vi "CCD photon image_Shaowei-v3.vi"() -> ()   [LabVIEW 2009]
uses:
  <vilib>/Utility/file.llb/Read From Spreadsheet File (DBL).vi
  Instance           5 35Saved   CCD photon image_540_800_CR .vi
  Instance           4 35Saved   CCD photon image_540_800_CR .vi
  Instance           3 35Saved   CCD photon image_540_800_CR .vi
  Instance           8 35Saved   CCD photon image_540_800_CR .vi
  <vilib>/Analysis/Matrix/Numeric/Conversions/Array To Matrix - RA2.vi
  Instance          12 35Saved   CCD photon image_540_800_CR .vi
  Instance          18 35Saved   CCD photon image_540_800_CR .vi
  <vilib>/Analysis/Matrix/NI_Matrix.lvlib
panel:
  in  "Full Range 5":bool caption="Full Range"
  in  "Full Range 4":bool caption="Full Range"
  in  "Full Range":bool
  in  "Full Range 3":bool caption="Full Range"
  in  "Full Range":bool
  in  "Full Range":bool
  in  "Save Matrix6":bool
  in  "Save Matrix5":bool
  in  "Save Matrix3":bool
  in  "Save Matrix4":bool
  out "Save As":string
  in  "Save Matrix2":bool
  out "Save As":string
  in  "Save Matrix1":bool
  in  "select 2":bool
  in  "select":bool
  in  "next 2":bool
  in  "next":bool
  in  "previous 2":bool
  in  "previous":bool
  in  "Do it":bool
  out "?":path
  out "?":path
  out "?":i32
  in  "?":bool
  in  "stop 2":bool
  in  "#6":bool
  in  "#5":bool
  in  "to":dbl=950.0
  in  "From":dbl=550.0
  out "Intensity Graph 6":dbl[][](graph)
  out "px":dbl
  out "px":dbl
  out "Save As":string
  in  "From 5":dbl caption="From"
  in  "To 5":dbl caption="To"
  out "eV":dbl format="%#_4g"
  out "eV":dbl format="%#_4g"
  out "Intensity Graph 5":dbl[][](graph)
  out "px":dbl
  out "px":dbl
  out "Save As":string
  in  "From 4":dbl caption="From"
  in  "To 4":dbl caption="To"
  out "eV":dbl format="%#_4g"
  out "eV":dbl format="%#_4g"
  in  "?":bool
  out "MAX":dbl
  out "MIN":dbl
  out "X":sgl
  out "Y":sgl
  out "px":dbl
  out "px":dbl
  out "eV":dbl format="%#_4g"
  out "eV":dbl format="%#_4g"
  in  "To 3":dbl caption="To"
  in  "From 3":dbl caption="From"
  out "eV":dbl format="%#_4g"
  out "eV":dbl format="%#_4g"
  in  "To":dbl
  in  "From":dbl
  out "px":dbl
  out "px":dbl
  out "px":dbl
  out "px":dbl
  out "eV":dbl format="%#_4g"
  out "eV":dbl format="%#_4g"
  in  "To":dbl
  in  "From":dbl
  in  "?":dbl=32.0
  out "eV":dbl format="%#_4g"
  out "eV":dbl format="%#_4g"
  in  "To":dbl
  in  "From":dbl
  out "px":dbl
  out "px":dbl
  in  "#3":bool
  in  "#4":bool
  in  "#2":bool
  out "Intensity Graph 4":dbl[][](graph)
  out "Save As":string
  out "Intensity Graph 3":dbl[][](graph)
  out "Save As":string
  out "Intensity Graph 2":dbl[][](graph)
  out "Intensity Graph":dbl[][](graph)
  # "Input File"
  # "nm"
  # "nm"
  # "nm"
  # "2 Files"
  # "1 File"
  # "nm"
  # "nm"
  # "nm"
  # "1st"
  # "2nd"
  # "Spectra Range"
  # "nm"
  # "nm"
  # "# of Pixel"
  # "Image Size"
  # "Bit"
  # "Active Window"
  # "nm"
  # "nm"
  # "nm"
  # "nm"
  # "nm"
  # "nm"
  # "Cosmic Ray Removal"
  # "NO"
  # "YES"
  # "Value"
  # "Position"
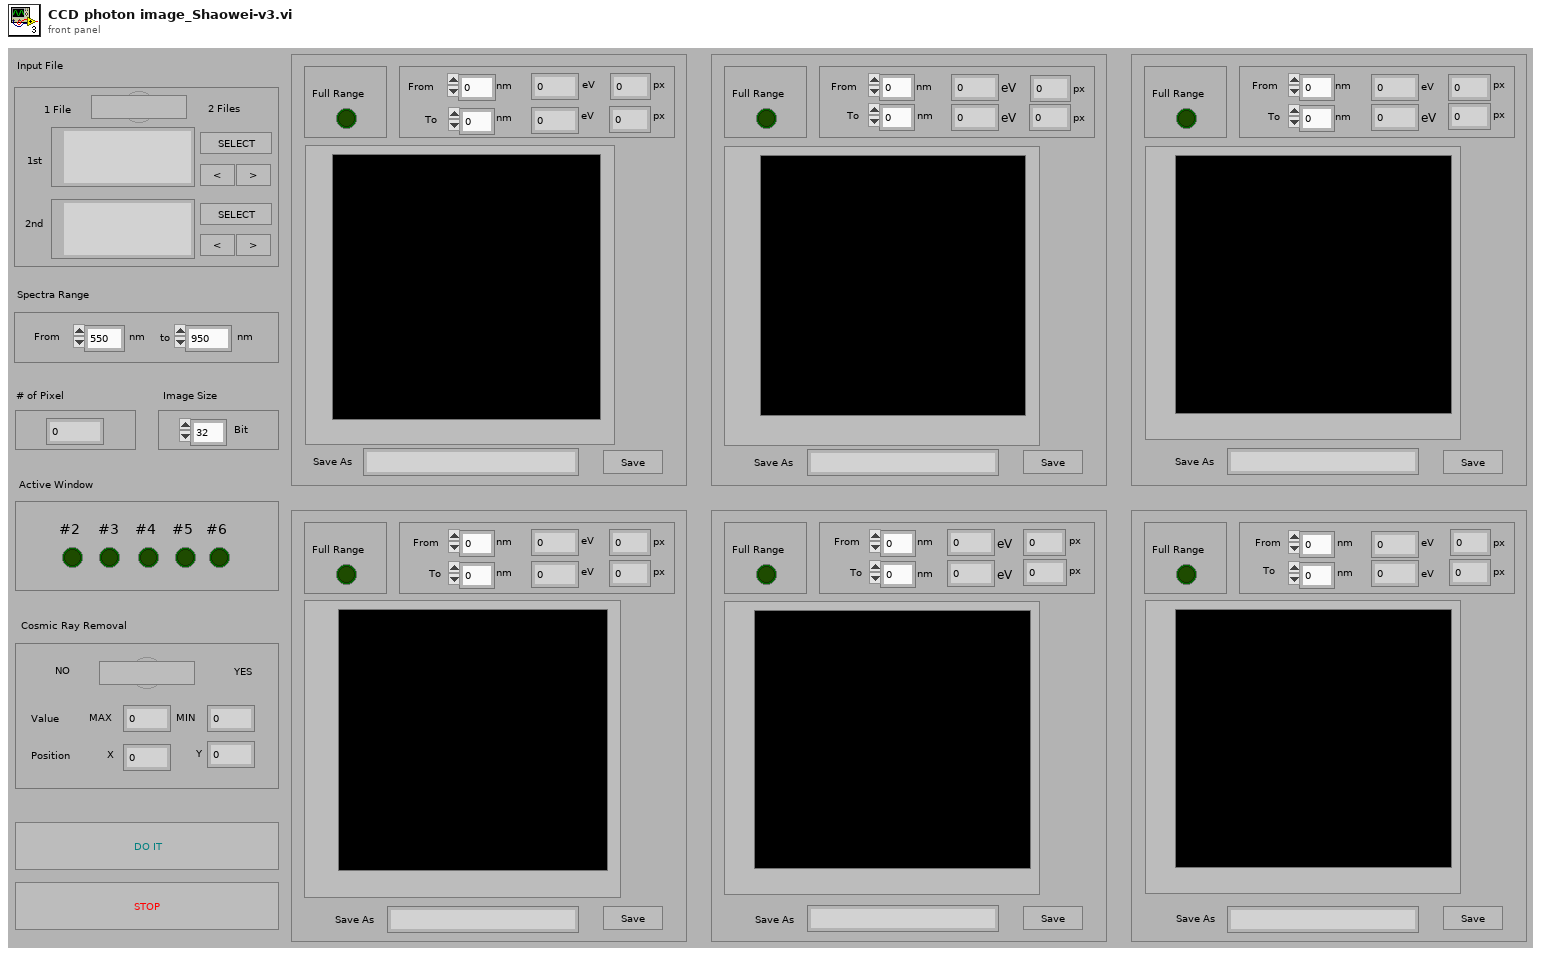
[diagram p1: front panel]
types:
  T1 = typedef "NI_Matrix.lvlib/RealMatrix.ctl" = dbl[][]
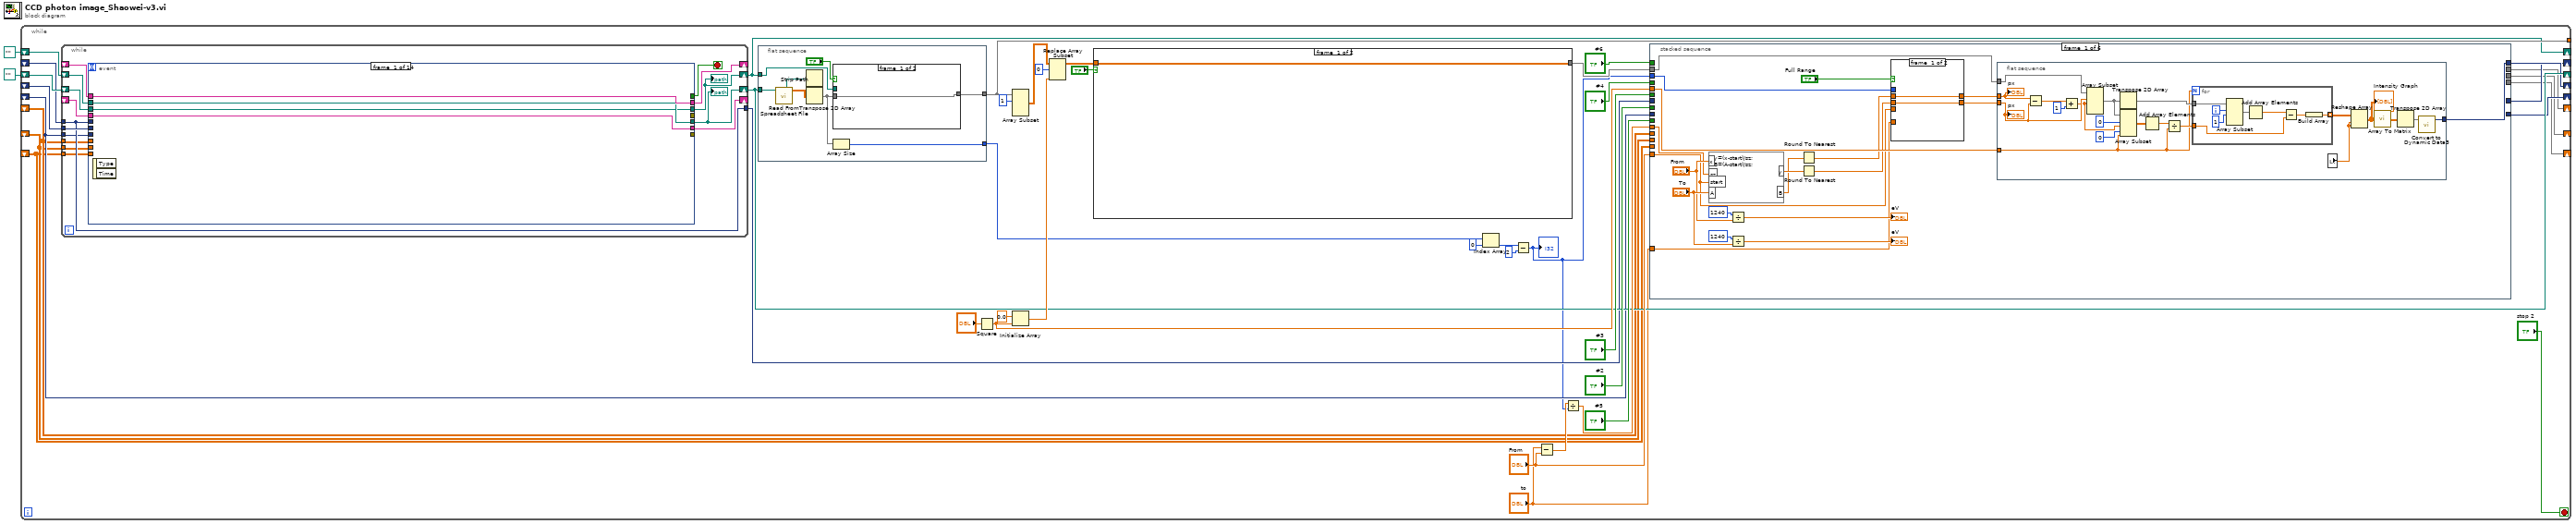
[diagram p0: block diagram]
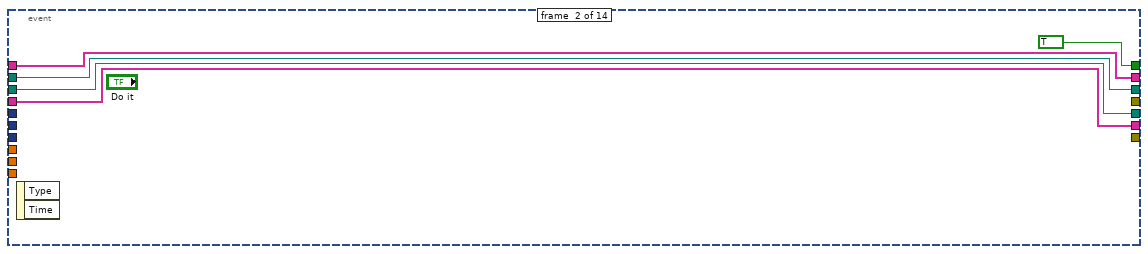
[diagram p2: hidden frame]
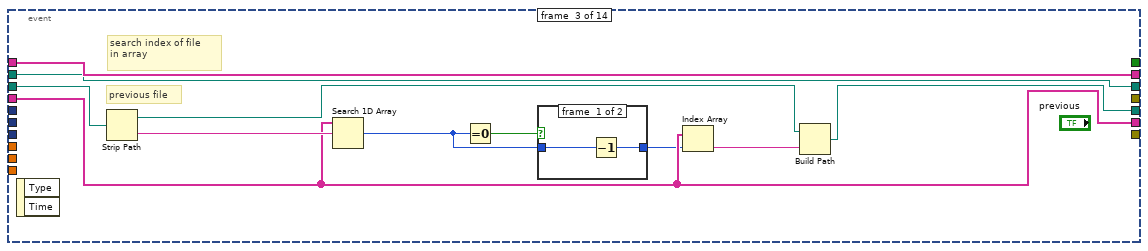
[diagram p3: hidden frame]
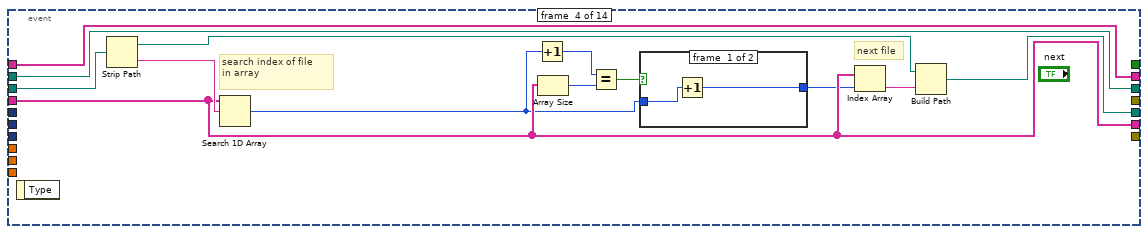
[diagram p5: hidden frame]
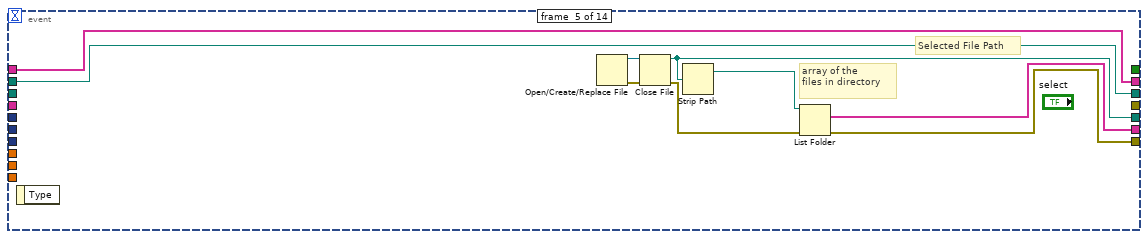
[diagram p7: hidden frame]
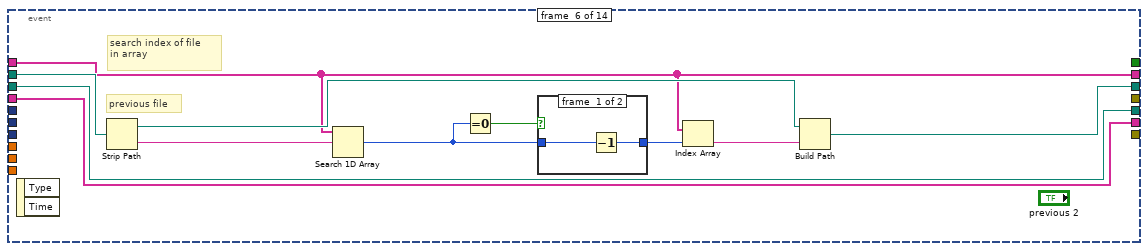
[diagram p8: hidden frame]
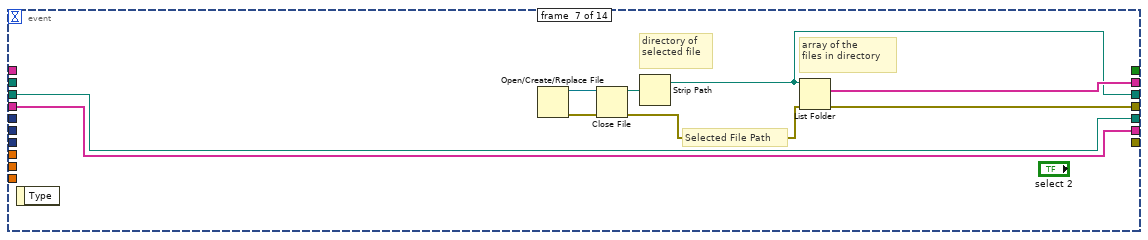
[diagram p10: hidden frame]
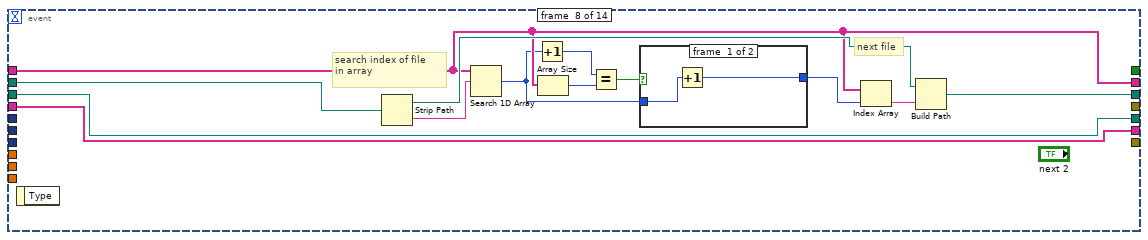
[diagram p11: hidden frame]
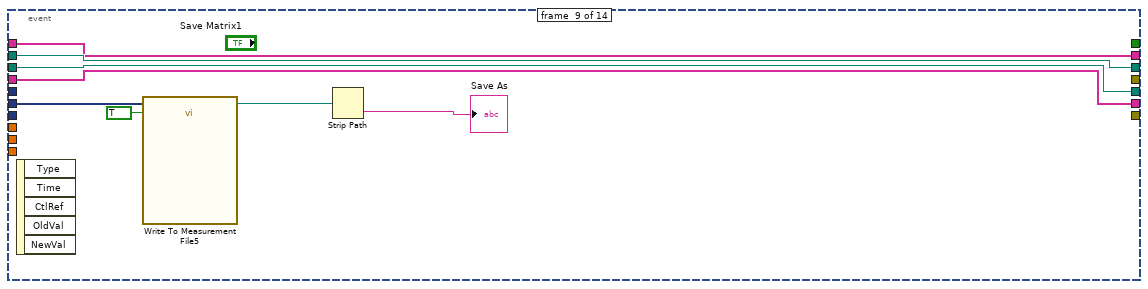
[diagram p13: hidden frame]
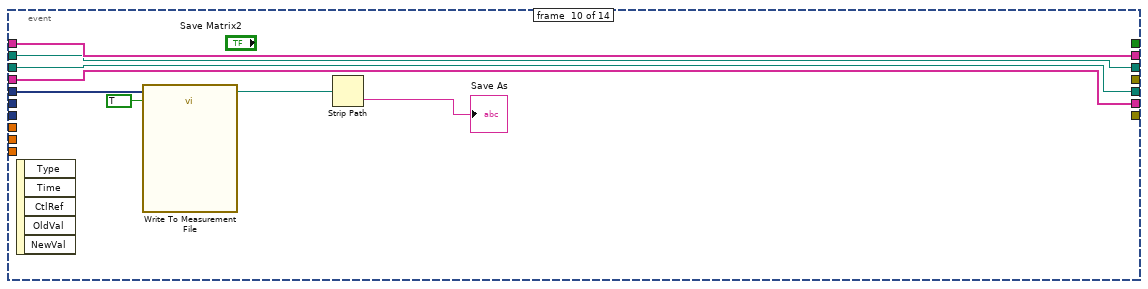
[diagram p14: hidden frame]
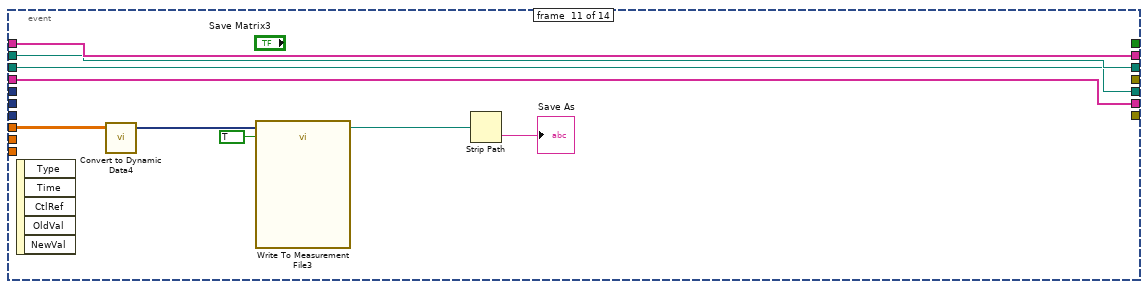
[diagram p15: hidden frame]
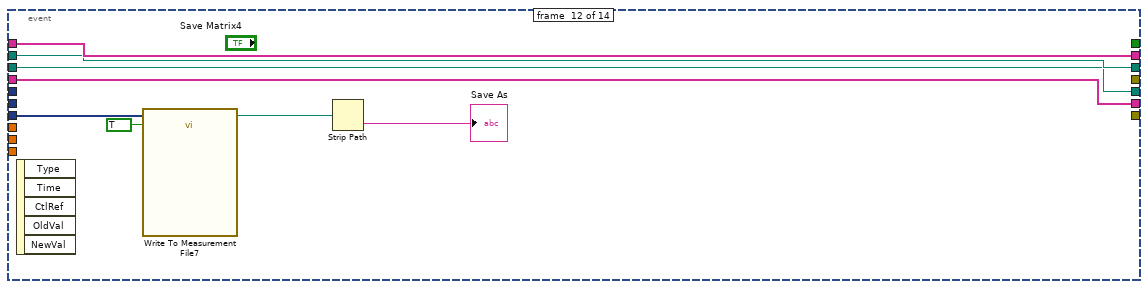
[diagram p16: hidden frame]
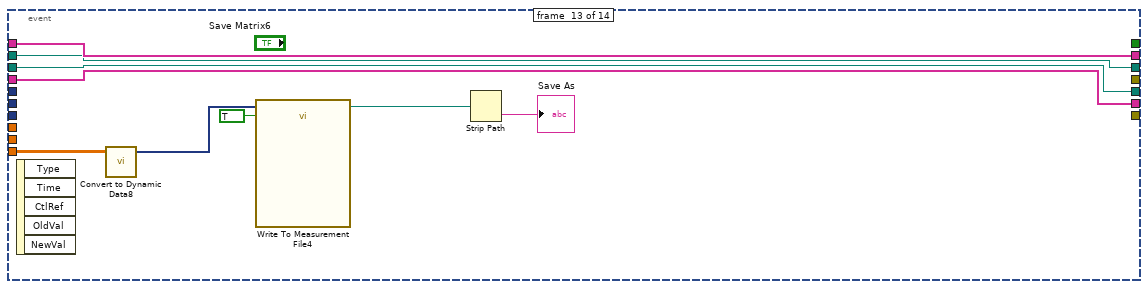
[diagram p17: hidden frame]
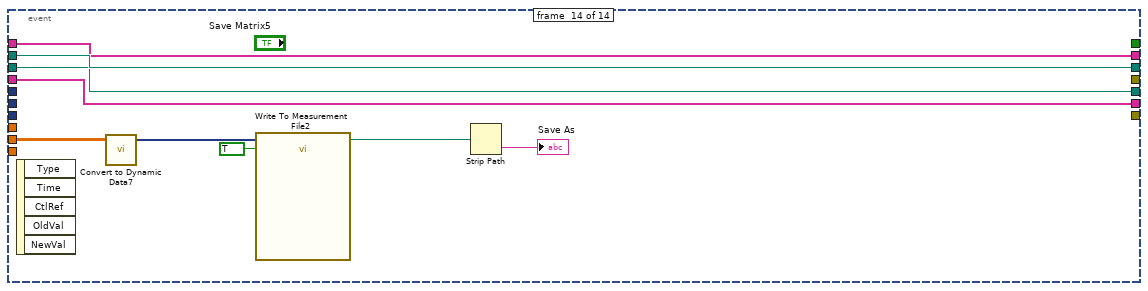
[diagram p18: hidden frame]
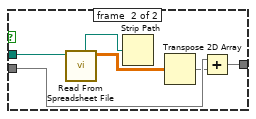
[diagram p19: hidden frame]
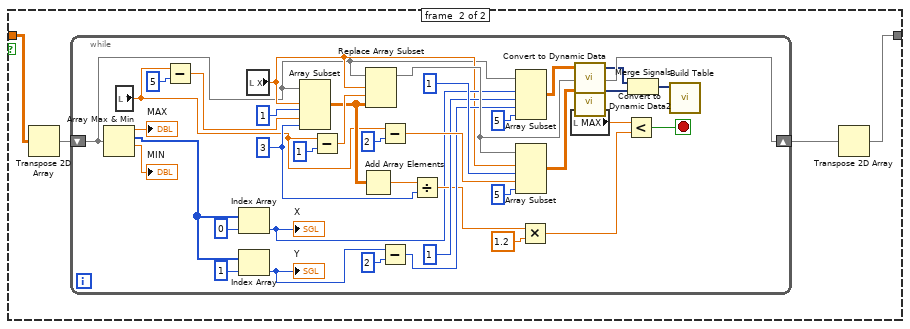
[diagram p20: hidden frame]
diagram:
  n1 = while {
    tunnel: [w27] -> _
    shift-right: [w18] -> _
    shift-left: path "" ("path") -> [w20]
    shift-right: [w19] -> _
    shift-left: path "" ("path") -> [w21]
    shift-right: [w17] -> _
    shift-left: _ -> [w16]
    shift-right: [w15] -> _
    shift-left: _ -> [w14]
    shift-right: [w12] -> _
    shift-left: _ -> [w11]
    shift-right: [w10] -> _
    shift-left: _ -> [w9]
    shift-right: [w8] -> _
    shift-left: _ -> [w7]
    shift-right: [w6] -> _
    shift-left: _ -> [w5]
    stop <- "stop 2" stop-if-true
    n2 = while {
      shift-right: [w60] -> _
      shift-left: _ -> [w59]
      shift-right: [w46] -> w18
      shift-left: w20 -> [w58]
      shift-right: [w47] -> w19
      shift-left: w21 -> [w57]
      shift-right: [w56] -> _
      shift-left: _ -> [w55]
      tunnel: w16 -> [w53]
      tunnel: w14 -> [w52]
      tunnel: [w52] -> w13
      tunnel: w11 -> [w51]
      tunnel: w9 -> [w50]
      tunnel: w7 -> [w49]
      tunnel: w5 -> [w48]
      stop <- w54 stop-if-true
      n3 = event shown="[1] \"Do it\": Value Change" {
        selector: _ -> [_ _ _ _ _ _ _ _ _ _ _ _ _ _]
        dyn-events: _ -> [_ _ _ _ _ _ _ _ _ _ _ _ _ _]
        timeout: _ -> [_ _ _ _ _ _ _ _ _ _ _ _ _ _]
        tunnel: [_ TRUE _ _ _ _ _ _ _ _ _ _ _ _] -> w54
        tunnel: [w63 w68 w75 w93 w103 w109 w130 w139 w151 w157 w165 w174 w182 w190] -> w46
        tunnel: [w64 w69 w77 w89 w107 w114 w129 w138 w148 w156 w164 w173 w181 w191] -> w60
        tunnel: w59 -> [w64 w69 w77 w89 _ w114 w129 w138 w148 w156 w164 w173 w181 w191]
        tunnel: w58 -> [w63 w68 w80 w92 _ w109 w130 w139 w151 w157 w165 w174 w182 w190]
        tunnel: [w61 w66 w73 w90 w105 w110 w128 w140 w150 w158 w166 w175 w183 w193] -> w47
        tunnel: w57 -> [w61 w66 w73 w90 w105 w116 _ w141 w150 w158 w166 w175 w183 w193]
        tunnel: [w62 w67 w74 w91 w106 w115 w131 w134 w149 w159 w167 w176 w184 w192] -> w56
        tunnel: w55 -> [w62 w67 w74 w91 w106 w115 _ w134 w149 w159 w167 w176 w184 w192]
        tunnel: w53 -> [_ _ _ _ _ _ _ _ w155 _ _ _ _ _]
        tunnel: w52 -> [_ _ _ _ _ _ _ _ _ w163 _ _ _ _]
        tunnel: w51 -> [_ _ _ _ _ _ _ _ _ _ _ w177 _ _]
        tunnel: w50 -> [_ _ _ _ _ _ _ _ _ _ w169 _ _ _]
        tunnel: w49 -> [_ _ _ _ _ _ _ _ _ _ _ _ _ w196]
        tunnel: w48 -> [_ _ _ _ _ _ _ _ _ _ _ _ w186 _]
        tunnel: [_ _ _ _ _ _ w123 _ _ _ _ _ _ _] -> _
        tunnel: [_ _ _ _ w100 _ _ _ _ _ _ _ _ _] -> _
        event #0 {
          n4 = event-data() -> ()  [unwired: 1 in, 2 out]
        }
        event #1 {
          n5 = event-data() -> ()  [unwired: 1 in, 2 out]
        }
        event #2 {
          # "previous file"
          # "search index of file\nin array"
          n6 = event-data() -> ()  [unwired: 1 in, 2 out]
          n7 = Strip Path(path=w80) -> (stripped path=w78:path, name=w79:string)
          n8 = Search 1D Array(1D array=w77, element=w79) -> (index of element=w71:i32)  [unwired: 1 in]
          n9 = Equal To 0?(x=w71) -> (x = 0?=w72:bool)
          n10 = case shown="False" w72 {
            tunnel: w71 -> [w82 w83]
            tunnel: [w81 w83] -> w70
            frame #0 {
              n11 = Decrement(x=w82) -> (x-1=w81:i32)
            }
            frame #1 {
            }
          }
          n12 = Index Array(array=w77, index=w70) -> (element=w76:string)
          n13 = Build Path(base path=w78, name or relative path=w76) -> (appended path=w75:path)
        }
        event #3 {
          # "next file"
          # "search index of file\nin array"
          n14 = event-data() -> ()  [unwired: 1 in, 1 out]
          n15 = Strip Path(path=w92) -> (stripped path=w95:path, name=w96:string)
          n16 = Search 1D Array(1D array=w89, element=w96) -> (index of element=w84:i32)  [unwired: 1 in]
          n17 = Increment(x=w84) -> (x+1=w85:i32)
          n18 = Array Size(array=w89) -> (size(s)=w88:i32)
          n19 = Equal?(x=w85, y=w88) -> (x = y?=w87:bool)
          n20 = case shown="True" w87 {
            tunnel: w84 -> [w98 w99]
            tunnel: [w97 w99] -> w86
            frame #0 {
              n21 = Increment(x=w98) -> (x+1=w97:i32)
            }
            frame #1 {
            }
          }
          n22 = Index Array(array=w89, index=w86) -> (element=w94:string)
          n23 = Build Path(base path=w95, name or relative path=w94) -> (appended path=w93:path)
        }
        event #4 {
          # "array of the \nfiles in directory"
          # "Selected File Path"
          n24 = event-data() -> ()  [unwired: 1 in, 1 out]
          n25 = Open/Create/Replace File() -> (refnum out=w104:refnum<file>, error out=w102:errorcluster)  [unwired: 6 in, 1 out]
          n26 = Close File(refnum=w104, error in=w102) -> (path=w103:path, error out=w101:errorcluster)
          n27 = Strip Path(path=w103) -> (stripped path=w108:path)  [unwired: 1 out]
          n28 = List Folder(path=w108, error in=w101) -> (filenames=w107:string[], error out=w100:errorcluster)  [unwired: 2 in, 2 out]
        }
        event #5 {
          # "previous file"
          # "search index of file\nin array"
          n29 = event-data() -> ()  [unwired: 1 in, 2 out]
          n30 = Strip Path(path=w116) -> (stripped path=w118:path, name=w119:string)
          n31 = Search 1D Array(1D array=w115, element=w119) -> (index of element=w112:i32)  [unwired: 1 in]
          n32 = Equal To 0?(x=w112) -> (x = 0?=w113:bool)
          n33 = case shown="False" w113 {
            tunnel: w112 -> [w121 w122]
            tunnel: [w120 w122] -> w111
            frame #0 {
              n34 = Decrement(x=w121) -> (x-1=w120:i32)
            }
            frame #1 {
            }
          }
          n35 = Index Array(array=w115, index=w111) -> (element=w117:string)
          n36 = Build Path(base path=w118, name or relative path=w117) -> (appended path=w110:path)
        }
        event #6 {
          # "array of the \nfiles in directory"
          # "directory of\nselected file"
          # "Selected File Path"
          n37 = event-data() -> ()  [unwired: 1 in, 1 out]
          n38 = Open/Create/Replace File() -> (refnum out=w127:refnum<file>, error out=w125:errorcluster)  [unwired: 6 in, 1 out]
          n39 = Close File(refnum=w127, error in=w125) -> (path=w126:path, error out=w124:errorcluster)
          n40 = Strip Path(path=w126) -> (stripped path=w128:path)  [unwired: 1 out]
          n41 = List Folder(path=w128, error in=w124) -> (filenames=w131:string[], error out=w123:errorcluster)  [unwired: 2 in, 2 out]
        }
        event #7 {
          # "next file"
          # "search index of file\nin array"
          n42 = event-data() -> ()  [unwired: 1 in, 1 out]
          n43 = Strip Path(path=w141) -> (stripped path=w143:path, name=w144:string)
          n44 = Search 1D Array(1D array=w134, element=w144) -> (index of element=w133:i32)  [unwired: 1 in]
          n45 = Increment(x=w133) -> (x+1=w135:i32)
          n46 = Array Size(array=w134) -> (size(s)=w137:i32)
          n47 = Equal?(x=w135, y=w137) -> (x = y?=w136:bool)
          n48 = case shown="True" w136 {
            tunnel: w133 -> [w146 w147]
            tunnel: [w145 w147] -> w132
            frame #0 {
              n49 = Increment(x=w146) -> (x+1=w145:i32)
            }
            frame #1 {
            }
          }
          n50 = Index Array(array=w134, index=w132) -> (element=w142:string)
          n51 = Build Path(base path=w143, name or relative path=w142) -> (appended path=w140:path)
        }
        event #8 {
          n52 = event-data() -> ()  [unwired: 1 in, 5 out]
          n53 = call "Write To Measurement File5"("Signals"=w155, "Reset"=TRUE) -> ("Filename Out"=w153:path)  [unwired: 15 in, 2 out]
          n54 = Strip Path(path=w153) -> (name=→"Save As":string)  [unwired: 1 out]
        }
        event #9 {
          n55 = event-data() -> ()  [unwired: 1 in, 5 out]
          n56 = call "Write To Measurement File"("Signals"=w163, "Reset"=TRUE) -> ("Filename Out"=w161:path)  [unwired: 15 in, 2 out]
          n57 = Strip Path(path=w161) -> (name=→"Save As":string)  [unwired: 1 out]
        }
        event #10 {
          n58 = event-data() -> ()  [unwired: 1 in, 5 out]
          n59 = call "Convert to Dynamic Data4"("2D Array"=w169) -> ("Dynamic Data Type"=w168:dynamicdata)  [unwired: 3 in]
          n60 = call "Write To Measurement File3"("Signals"=w168, "Reset"=TRUE) -> ("Filename Out"=w172:path)  [unwired: 15 in, 2 out]
          n61 = Strip Path(path=w172) -> (name=→"Save As":string)  [unwired: 1 out]
        }
        event #11 {
          n62 = event-data() -> ()  [unwired: 1 in, 5 out]
          n63 = call "Write To Measurement File7"("Signals"=w177, "Reset"=TRUE) -> ("Filename Out"=w179:path)  [unwired: 15 in, 2 out]
          n64 = Strip Path(path=w179) -> (name=→"Save As":string)  [unwired: 1 out]
        }
        event #12 {
          n65 = event-data() -> ()  [unwired: 1 in, 5 out]
          n66 = call "Convert to Dynamic Data8"("2D Array"=w186) -> ("Dynamic Data Type"=w185:dynamicdata)  [unwired: 3 in]
          n67 = call "Write To Measurement File4"("Signals"=w185, "Reset"=TRUE) -> ("Filename Out"=w188:path)  [unwired: 15 in, 2 out]
          n68 = Strip Path(path=w188) -> (name=→"Save As":string)  [unwired: 1 out]
        }
        event #13 {
          n69 = event-data() -> ()  [unwired: 1 in, 5 out]
          n70 = call "Convert to Dynamic Data7"("2D Array"=w196) -> ("Dynamic Data Type"=w195:dynamicdata)  [unwired: 3 in]
          n71 = call "Write To Measurement File2"("Signals"=w195, "Reset"=TRUE) -> ("Filename Out"=w197:path)  [unwired: 15 in, 2 out]
          n72 = Strip Path(path=w197) -> (name=→"Save As":string)  [unwired: 1 out]
        }
      }
      "?" <- w46
      "?" <- w47
    }
    n73 = flat-sequence {
      tunnel: [w205] -> w27
      tunnel: [w202] -> w25
      tunnel: w18 -> [w200]
      tunnel: w19 -> [w199]
      frame #0 {
        n74 = call-poly <vilib>:"Read From Spreadsheet File.vi"("file path (dialog if empty)"=w200) -> ("all rows"=w203:dbl[][], "new file path (Not A Path if cancelled)"=w206:path)  [unwired: 6 in, 3 out]
        n75 = Strip Path(path=w206) -> ()  [unwired: 2 out]
        n76 = Transpose 2D Array(2D array=w203) -> (transposed array=w201:dbl[][])
        n77 = case shown="True" "?" {
          tunnel: w201 -> [w207 w212]
          tunnel: [w207 w211] -> w205
          tunnel: w199 -> [_ w208]
          frame #0 {
          }
          frame #1 {
            n78 = call-poly <vilib>:"Read From Spreadsheet File.vi"("file path (dialog if empty)"=w208) -> ("all rows"=w210:dbl[][], "new file path (Not A Path if cancelled)"=w213:path)  [unwired: 6 in, 3 out]
            n79 = Strip Path(path=w213) -> ()  [unwired: 2 out]
            n80 = Transpose 2D Array(2D array=w210) -> (transposed array=w209:dbl[][])
            n81 = Add(x=w212, y=w209) -> (x+y=w211:dbl[][])
          }
        }
        n82 = Array Size(array=w201) -> (size(s)=w202:i32[])
      }
    }
    n83 = Square(x="?") -> (x^2=w37:dbl)
    n84 = Array Subset(array=w27, index (row)=1) -> (w39:dbl[][])  [unwired: 3 in]
    n85 = Initialize Array(0.0 ("element"), w37) -> (w41:dbl[])
    n86 = Replace Array Subset(array=w39, new element=w41, index (row)=0) -> (w36:dbl[][])  [unwired: 1 in]
    n87 = case shown="True" "?" {
      tunnel: w36 -> [w214 w218]
      tunnel: [w214 w216] -> w35
      frame #0 {
      }
      frame #1 {
        n88 = Transpose 2D Array(2D array=w218) -> (transposed array=w217:dbl[][])
        n89 = while {
          shift-right: [w255] -> w215
          shift-left: w217 -> [w219]
          stop <- w234 stop-if-true
          w232 = 3
          n90 = Array Max & Min(array=w219) -> (max value=→"MAX":dbl, max index (indices)=w253:i32[], min value=→"MIN":dbl)  [unwired: 1 out]
          n91 = local read "Y"() -> (w221:sgl)
          n92 = Subtract(x=w221, y=5) -> (x-y=w249:sgl)
          n93 = Index Array(array=w253, index=0) -> (element=w226:i32)
          "X" <- w226
          n94 = Index Array(array=w253, index=1) -> (element=w225:i32)
          "Y" <- w225
          n95 = local read "X"() -> (w222:sgl)
          n96 = Array Subset(array=w219, index (row)=w222, length (row)=1, index (col)=w249, length (col)=w232) -> (w231:dbl[][])
          n97 = Subtract(x=w221, y=1) -> (x-y=w248:sgl)
          n98 = Add Array Elements(numeric array=w231) -> (sum=w233:dbl)
          n99 = Replace Array Subset(array=w219, new element=w231, index (row)=w222, index (col)=w248) -> (w255:dbl[][])
          n100 = Subtract(x=w221, y=2) -> (x-y=w244:sgl)
          n101 = Subtract(x=w225, y=2) -> (x-y=w239:i32)
          n102 = Divide(x=w233, y=w232) -> (x/y=w230:dbl)
          n103 = Array Subset(array=w219, index (row)=w226, length (row)=1, index (col)=w239, length (col)=5) -> (w237:dbl[][])
          n104 = Array Subset(array=w255, index (row)=w222, length (row)=1, index (col)=w244, length (col)=5) -> (w242:dbl[][])
          n105 = Multiply(x=w230, y=1.2) -> (x*y=w235:dbl)
          n106 = local read "MAX"() -> (w220:dbl)
          n107 = call "Convert to Dynamic Data"("2D Array"=w237) -> ("Dynamic Data Type"=w229:dynamicdata)  [unwired: 3 in]
          n108 = call "Convert to Dynamic Data2"("2D Array"=w242) -> ("Dynamic Data Type"=w227:dynamicdata)  [unwired: 3 in]
          n109 = Less?(x=w220, y=w235) -> (x < y?=w234:bool)
          n110 = Merge Signals(w229, w227) -> (w228:dynamicdata)
          n111 = call "Build Table"("Signals"=w228) -> ()  [unwired: 9 in, 2 out]
        }
        n112 = Transpose 2D Array(2D array=w215) -> (transposed array=w216:dbl[][])
      }
    }
    n113 = Index Array(array=w25, index=0) -> (element=w23:i32)
    n114 = Subtract(x=w23, y=2) -> (x-y=w4:i32)
    "?" <- w4
    n115 = Subtract(x="to", y="From") -> (x-y=w33:dbl)
    n116 = Divide(x=w33, y=w4) -> (x/y=w32:dbl)
    n117 = stacked-sequence {
      tunnel: "#4" -> [_ _ _ w445 _ _]
      tunnel: "#3" -> [_ _ w382 _ _ _]
      tunnel: "#2" -> [_ w318 _ _ _ _]
      tunnel: w37 -> [w267 w317 w381 w437 w503 w566]
      tunnel: w35 -> [w266 w316 w380 w444 w509 w572]
      tunnel: w32 -> [w265 w315 w379 w442 w508 w571]
      tunnel: "From" -> [w257 w314 w378 w443 w507 w570]
      tunnel: "#5" -> [_ _ _ _ w506 _]
      tunnel: "#6" -> [_ _ _ _ _ w569]
      tunnel: [w264 _ _ _ _ _] -> w17
      tunnel: [_ w313 _ _ _ _] -> w15
      tunnel: w13 -> [_ w312 _ _ _ _]
      tunnel: [_ _ _ w441 _ _] -> w12
      tunnel: w11 -> [_ _ _ w440 _ _]
      tunnel: [_ _ w377 _ _ _] -> w10
      tunnel: w9 -> [_ _ w376 _ _ _]
      tunnel: [_ _ _ _ w505 _] -> w8
      tunnel: w7 -> [_ _ _ _ w504 _]
      tunnel: [_ _ _ _ _ w568] -> w6
      tunnel: w5 -> [_ _ _ _ _ w567]
      tunnel: w4 -> [w258 w310 w374 w438 w502 w564]
      tunnel: "to" -> [w256 w311 w375 w439 w501 w565]
      frame #0 {
        n118 = formula code="y=(x-start)/sz;\nB=(A-start)/sz;"("x"="From", "A"="To", "sz"=w265, "start"=w257) -> ("y"=w269:dbl, "B"=w268:dbl)
        n119 = Divide(x=1240, y="From") -> (x/y=→"eV":dbl)
        n120 = Divide(x=1240, y="To") -> (x/y=→"eV":dbl)
        n121 = Round To Nearest(number=w268) -> (nearest integer value=w262:dbl)
        n122 = Round To Nearest(number=w269) -> (nearest integer value=w260:dbl)
        n123 = case shown="False" "Full Range" {
          tunnel: w262 -> [w277 _]
          tunnel: [w277 w278] -> w261
          tunnel: w260 -> [w276 _]
          tunnel: [w276 0.0] -> w259
          tunnel: w258 -> [_ w278]
          tunnel: w257 -> [_ w281]
          tunnel: w256 -> [_ w280]
          frame #0 {
          }
          frame #1 {
            n124 = local write "From"(w281) -> ()
            n125 = local write "To"(w280) -> ()
          }
        }
        n126 = flat-sequence {
          tunnel: [w301] -> w264
          tunnel: w261 -> [w294]
          tunnel: w259 -> [w293]
          tunnel: w267 -> [w282]
          tunnel: w266 -> [w286]
          frame #0 {
            n127 = Subtract(x=w294, y=w293) -> (x-y=w289:dbl)
            n128 = Add(x=w289, y=1) -> (x+y=w287:dbl)
            n129 = Array Subset(array=w286, index (row)=w293, length (row)=w287) -> (w285:dbl[][])  [unwired: 2 in]
            n130 = Transpose 2D Array(2D array=w285) -> (transposed array=w296:dbl[][])
            n131 = Array Subset(array=w285, index (row)=0, length (row)=w287, index (col)=0, length (col)=w282) -> (w284:dbl[][])
            n132 = Add Array Elements(numeric array=w284) -> (sum=w290:dbl)
            n133 = Divide(x=w290, y=w282) -> (x/y=w288:dbl)
            n134 = for {
              N: w282 -> [_]
              tunnel: w296 -> [w303]
              tunnel: [w305] -> w295 mode=indexing
              tunnel: w288 -> [w304]
              i -> [w309]
              n135 = Array Subset(array=w303, index (row)=w309, length (row)=1) -> (w302:dbl[][])  [unwired: 2 in]
              n136 = Add Array Elements(numeric array=w302) -> (sum=w307:dbl)
              n137 = Subtract(x=w307, y=w304) -> (x-y=w306:dbl)
              n138 = Build Array(w306) -> (w305:dbl[])
            }
            n139 = local read item#15() -> (w283:dbl)
            n140 = Reshape Array(w295, w283, w283) -> (w297:dbl[][])
            "Intensity Graph" <- w297
            n141 = call-poly <vilib>:"Array To Matrix.vi"("Real 2D Array"=w297) -> ("Real Matrix"=w300:T1)
            n142 = Transpose 2D Array(2D array=w300) -> (transposed array=w299:T1)
            n143 = call "Convert to Dynamic Data3"("2D Array"=w299) -> ("Dynamic Data Type"=w301:dynamicdata)  [unwired: 3 in]
            "px" <- w293
            "px" <- w294
          }
        }
      }
      frame #1 {
        n144 = case shown="True" w318 {
          tunnel: w317 -> [_ w332]
          tunnel: w316 -> [_ w331]
          tunnel: w315 -> [_ w330]
          tunnel: w314 -> [_ w323]
          tunnel: [w319 w328] -> w313
          tunnel: w312 -> [w319 _]
          tunnel: w311 -> [_ w322]
          tunnel: w310 -> [_ w321]
          frame #0 {
          }
          frame #1 {
            n145 = formula code="y=(x-start)/sz;\nB=(A-start)/sz;"("x"="From", "A"="To", "sz"=w330, "start"=w323) -> ("y"=w334:dbl, "B"=w333:dbl)
            n146 = Divide(x=1240, y="From") -> (x/y=→"eV":dbl)
            n147 = Divide(x=1240, y="To") -> (x/y=→"eV":dbl)
            n148 = Round To Nearest(number=w333) -> (nearest integer value=w325:dbl)
            n149 = Round To Nearest(number=w334) -> (nearest integer value=w327:dbl)
            n150 = case shown="True" "Full Range" {
              tunnel: w325 -> [w342 _]
              tunnel: [w342 w345] -> w324
              tunnel: w327 -> [w341 _]
              tunnel: [w341 0.0] -> w326
              tunnel: w321 -> [_ w345]
              tunnel: w323 -> [_ w344]
              tunnel: w322 -> [_ w343]
              frame #0 {
              }
              frame #1 {
                n151 = local write "From"(w344) -> ()
                n152 = local write "To"(w343) -> ()
              }
            }
            n153 = flat-sequence {
              tunnel: w326 -> [w352]
              tunnel: w324 -> [w353]
              tunnel: [w360] -> w329
              tunnel: w332 -> [w348]
              tunnel: w331 -> [w347]
              frame #0 {
                n154 = Subtract(x=w353, y=w352) -> (x-y=w361:dbl)
                n155 = Add(x=w361, y=1) -> (x+y=w355:dbl)
                n156 = Array Subset(array=w347, index (row)=w352, length (row)=w355) -> (w351:dbl[][])  [unwired: 2 in]
                n157 = Transpose 2D Array(2D array=w351) -> (transposed array=w364:dbl[][])
                n158 = Array Subset(array=w351, index (row)=0, length (row)=w355, index (col)=0, length (col)=w348) -> (w349:dbl[][])
                n159 = Add Array Elements(numeric array=w349) -> (sum=w358:dbl)
                n160 = Divide(x=w358, y=w348) -> (x/y=w354:dbl)
                n161 = for {
                  N: w348 -> [_]
                  tunnel: w364 -> [w373]
                  tunnel: [w366] -> w365 mode=indexing
                  tunnel: w354 -> [w368]
                  i -> [w372]
                  n162 = Array Subset(array=w373, index (row)=w372, length (row)=1) -> (w371:dbl[][])  [unwired: 2 in]
                  n163 = Add Array Elements(numeric array=w371) -> (sum=w369:dbl)
                  n164 = Subtract(x=w369, y=w368) -> (x-y=w367:dbl)
                  n165 = Build Array(w367) -> (w366:dbl[])
                }
                n166 = local read item#15() -> (w350:dbl)
                n167 = Reshape Array(w365, w350, w350) -> (w363:dbl[][])
                "Intensity Graph 2" <- w363
                n168 = call-poly <vilib>:"Array To Matrix.vi"("Real 2D Array"=w363) -> ("Real Matrix"=w359:T1)
                n169 = Transpose 2D Array(2D array=w359) -> (transposed array=w360:T1)
                "px" <- w352
                "px" <- w353
              }
            }
            n170 = call "Convert to Dynamic Data5"("2D Array"=w329) -> ("Dynamic Data Type"=w328:dynamicdata)  [unwired: 3 in]
          }
        }
      }
      frame #2 {
        n171 = case shown="True" w382 {
          tunnel: w381 -> [_ w395]
          tunnel: w380 -> [_ w394]
          tunnel: w379 -> [_ w393]
          tunnel: w378 -> [_ w391]
          tunnel: [w383 w392] -> w377
          tunnel: w376 -> [w383 _]
          tunnel: w375 -> [_ w389]
          tunnel: w374 -> [_ w384]
          frame #0 {
          }
          frame #1 {
            n172 = formula code="y=(x-start)/sz;\nB=(A-start)/sz;"("x"="From", "A"="To", "sz"=w393, "start"=w391) -> ("y"=w401:dbl, "B"=w400:dbl)
            n173 = Divide(x=1240, y="From") -> (x/y=→"eV":dbl)
            n174 = Divide(x=1240, y="To") -> (x/y=→"eV":dbl)
            n175 = Round To Nearest(number=w400) -> (nearest integer value=w386:dbl)
            n176 = Round To Nearest(number=w401) -> (nearest integer value=w388:dbl)
            n177 = case shown="True" "Full Range" {
              tunnel: [w405 0.0] -> w387
              tunnel: w391 -> [_ w409]
              tunnel: w389 -> [_ w407]
              tunnel: w388 -> [w405 _]
              tunnel: w386 -> [w404 _]
              tunnel: [w404 w406] -> w385
              tunnel: w384 -> [_ w406]
              frame #0 {
              }
              frame #1 {
                n178 = local write "From"(w409) -> ()
                n179 = local write "To"(w407) -> ()
              }
            }
            n180 = flat-sequence {
              tunnel: w385 -> [w415]
              tunnel: w387 -> [w416]
              tunnel: [w423] -> w392
              tunnel: w395 -> [w411]
              tunnel: w394 -> [w410]
              frame #0 {
                n181 = Subtract(x=w415, y=w416) -> (x-y=w424:dbl)
                n182 = Add(x=w424, y=1) -> (x+y=w418:dbl)
                n183 = Array Subset(array=w410, index (row)=w416, length (row)=w418) -> (w412:dbl[][])  [unwired: 2 in]
                n184 = Transpose 2D Array(2D array=w412) -> (transposed array=w427:dbl[][])
                n185 = Array Subset(array=w412, index (row)=0, length (row)=w418, index (col)=0, length (col)=w411) -> (w413:dbl[][])
                n186 = Add Array Elements(numeric array=w413) -> (sum=w419:dbl)
                n187 = Divide(x=w419, y=w411) -> (x/y=w417:dbl)
                n188 = for {
                  N: w411 -> [_]
                  tunnel: w427 -> [w436]
                  tunnel: [w430] -> w428 mode=indexing
                  tunnel: w417 -> [w429]
                  i -> [w435]
                  n189 = Array Subset(array=w436, index (row)=w435, length (row)=1) -> (w434:dbl[][])  [unwired: 2 in]
                  n190 = Add Array Elements(numeric array=w434) -> (sum=w432:dbl)
                  n191 = Subtract(x=w432, y=w429) -> (x-y=w431:dbl)
                  n192 = Build Array(w431) -> (w430:dbl[])
                }
                n193 = local read item#15() -> (w414:dbl)
                n194 = Reshape Array(w428, w414, w414) -> (w426:dbl[][])
                "Intensity Graph 3" <- w426
                n195 = call-poly <vilib>:"Array To Matrix.vi"("Real 2D Array"=w426) -> ("Real Matrix"=w422:T1)
                n196 = Transpose 2D Array(2D array=w422) -> (transposed array=w423:T1)
                "px" <- w416
                "px" <- w415
              }
            }
          }
        }
      }
      frame #3 {
        n197 = case shown="True" w445 {
          tunnel: w437 -> [_ w459]
          tunnel: w444 -> [_ w458]
          tunnel: w443 -> [_ w454]
          tunnel: w442 -> [_ w457]
          tunnel: [w446 w455] -> w441
          tunnel: w440 -> [w446 _]
          tunnel: w439 -> [_ w453]
          tunnel: w438 -> [_ w452]
          frame #0 {
          }
          frame #1 {
            n198 = formula code="y=(x-start)/sz;\nB=(A-start)/sz;"("x"="From 3", "A"="To 3", "sz"=w457, "start"=w454) -> ("y"=w465:dbl, "B"=w464:dbl)
            n199 = Divide(x=1240, y="To 3") -> (x/y=→"eV":dbl)
            n200 = Divide(x=1240, y="From 3") -> (x/y=→"eV":dbl)
            n201 = Round To Nearest(number=w464) -> (nearest integer value=w448:dbl)
            n202 = Round To Nearest(number=w465) -> (nearest integer value=w449:dbl)
            n203 = case shown="True" "Full Range 3" {
              tunnel: w448 -> [w469 _]
              tunnel: [w469 w473] -> w447
              tunnel: w449 -> [w468 _]
              tunnel: [w468 0.0] -> w450
              tunnel: w452 -> [_ w473]
              tunnel: w454 -> [_ w471]
              tunnel: w453 -> [_ w470]
              frame #0 {
              }
              frame #1 {
                n204 = local write "From 3"(w471) -> ()
                n205 = local write "To 3"(w470) -> ()
              }
            }
            n206 = flat-sequence {
              tunnel: w450 -> [w481]
              tunnel: w447 -> [w480]
              tunnel: [w488] -> w456
              tunnel: w459 -> [w474]
              tunnel: w458 -> [w475]
              frame #0 {
                n207 = Subtract(x=w480, y=w481) -> (x-y=w489:dbl)
                n208 = Add(x=w489, y=1) -> (x+y=w482:dbl)
                n209 = Array Subset(array=w475, index (row)=w481, length (row)=w482) -> (w479:dbl[][])  [unwired: 2 in]
                n210 = Transpose 2D Array(2D array=w479) -> (transposed array=w478:dbl[][])
                n211 = Array Subset(array=w479, index (row)=0, length (row)=w482, index (col)=0, length (col)=w474) -> (w476:dbl[][])
                n212 = Add Array Elements(numeric array=w476) -> (sum=w484:dbl)
                n213 = Divide(x=w484, y=w474) -> (x/y=w483:dbl)
                n214 = for {
                  N: w474 -> [_]
                  tunnel: w478 -> [w500]
                  tunnel: [w494] -> w492 mode=indexing
                  tunnel: w483 -> [w493]
                  i -> [w499]
                  n215 = Array Subset(array=w500, index (row)=w499, length (row)=1) -> (w498:dbl[][])  [unwired: 2 in]
                  n216 = Add Array Elements(numeric array=w498) -> (sum=w496:dbl)
                  n217 = Subtract(x=w496, y=w493) -> (x-y=w495:dbl)
                  n218 = Build Array(w495) -> (w494:dbl[])
                }
                n219 = local read item#15() -> (w477:dbl)
                n220 = Reshape Array(w492, w477, w477) -> (w491:dbl[][])
                "Intensity Graph 4" <- w491
                n221 = call-poly <vilib>:"Array To Matrix.vi"("Real 2D Array"=w491) -> ("Real Matrix"=w487:T1)
                n222 = Transpose 2D Array(2D array=w487) -> (transposed array=w488:T1)
                "px" <- w481
                "px" <- w480
              }
            }
            n223 = call "Convert to Dynamic Data6"("2D Array"=w456) -> ("Dynamic Data Type"=w455:dynamicdata)  [unwired: 3 in]
          }
        }
      }
      frame #4 {
        n224 = case shown="True" w506 {
          tunnel: w503 -> [_ w522]
          tunnel: w509 -> [_ w521]
          tunnel: w508 -> [_ w520]
          tunnel: w507 -> [_ w516]
          tunnel: [w510 w519] -> w505
          tunnel: w504 -> [w510 _]
          tunnel: w502 -> [_ w517]
          tunnel: w501 -> [_ w515]
          frame #0 {
          }
          frame #1 {
            n225 = formula code="y=(x-start)/sz;\nB=(A-start)/sz;"("x"="From 4", "A"="To 4", "sz"=w520, "start"=w516) -> ("y"=w528:dbl, "B"=w527:dbl)
            n226 = Divide(x=1240, y="From 4") -> (x/y=→"eV":dbl)
            n227 = Divide(x=1240, y="To 4") -> (x/y=→"eV":dbl)
            n228 = Round To Nearest(number=w527) -> (nearest integer value=w511:dbl)
            n229 = Round To Nearest(number=w528) -> (nearest integer value=w512:dbl)
            n230 = case shown="True" "Full Range 4" {
              tunnel: w511 -> [w532 _]
              tunnel: [w532 w536] -> w513
              tunnel: w512 -> [w531 _]
              tunnel: [w531 0.0] -> w514
              tunnel: w517 -> [_ w536]
              tunnel: w516 -> [_ w533]
              tunnel: w515 -> [_ w534]
              frame #0 {
              }
              frame #1 {
                n231 = local write "From 4"(w533) -> ()
                n232 = local write "To 4"(w534) -> ()
              }
            }
            n233 = flat-sequence {
              tunnel: w514 -> [w544]
              tunnel: w513 -> [w543]
              tunnel: [w551] -> w519
              tunnel: w522 -> [w537]
              tunnel: w521 -> [w538]
              frame #0 {
                n234 = Subtract(x=w543, y=w544) -> (x-y=w552:dbl)
                n235 = Add(x=w552, y=1) -> (x+y=w545:dbl)
                n236 = Array Subset(array=w538, index (row)=w544, length (row)=w545) -> (w542:dbl[][])  [unwired: 2 in]
                n237 = Transpose 2D Array(2D array=w542) -> (transposed array=w541:dbl[][])
                n238 = Array Subset(array=w542, index (row)=0, length (row)=w545, index (col)=0, length (col)=w537) -> (w539:dbl[][])
                n239 = Add Array Elements(numeric array=w539) -> (sum=w547:dbl)
                n240 = Divide(x=w547, y=w537) -> (x/y=w546:dbl)
                n241 = for {
                  N: w537 -> [_]
                  tunnel: w541 -> [w563]
                  tunnel: [w557] -> w555 mode=indexing
                  tunnel: w546 -> [w556]
                  i -> [w562]
                  n242 = Array Subset(array=w563, index (row)=w562, length (row)=1) -> (w561:dbl[][])  [unwired: 2 in]
                  n243 = Add Array Elements(numeric array=w561) -> (sum=w559:dbl)
                  n244 = Subtract(x=w559, y=w556) -> (x-y=w558:dbl)
                  n245 = Build Array(w558) -> (w557:dbl[])
                }
                n246 = local read item#15() -> (w540:dbl)
                n247 = Reshape Array(w555, w540, w540) -> (w554:dbl[][])
                "Intensity Graph 5" <- w554
                n248 = call-poly <vilib>:"Array To Matrix.vi"("Real 2D Array"=w554) -> ("Real Matrix"=w550:T1)
                n249 = Transpose 2D Array(2D array=w550) -> (transposed array=w551:T1)
                "px" <- w544
                "px" <- w543
              }
            }
          }
        }
      }
      frame #5 {
        n250 = case shown="True" w569 {
          tunnel: w566 -> [_ w585]
          tunnel: w572 -> [_ w584]
          tunnel: w571 -> [_ w583]
          tunnel: w570 -> [_ w581]
          tunnel: [w573 w582] -> w568
          tunnel: w567 -> [w573 _]
          tunnel: w565 -> [_ w580]
          tunnel: w564 -> [_ w577]
          frame #0 {
          }
          frame #1 {
            n251 = formula code="y=(x-start)/sz;\nB=(A-start)/sz;"("x"="From 5", "A"="To 5", "sz"=w583, "start"=w581) -> ("y"=w591:dbl, "B"=w590:dbl)
            n252 = Divide(x=1240, y="To 5") -> (x/y=→"eV":dbl)
            n253 = Divide(x=1240, y="From 5") -> (x/y=→"eV":dbl)
            n254 = Round To Nearest(number=w590) -> (nearest integer value=w575:dbl)
            n255 = Round To Nearest(number=w591) -> (nearest integer value=w576:dbl)
            n256 = case shown="False" "Full Range 5" {
              tunnel: w575 -> [w595 _]
              tunnel: [w595 w599] -> w578
              tunnel: w576 -> [w594 _]
              tunnel: [w594 0.0] -> w579
              tunnel: w577 -> [_ w599]
              tunnel: w581 -> [_ w596]
              tunnel: w580 -> [_ w597]
              frame #0 {
              }
              frame #1 {
                n257 = local write "From 5"(w596) -> ()
                n258 = local write "To 5"(w597) -> ()
              }
            }
            n259 = flat-sequence {
              tunnel: w579 -> [w607]
              tunnel: w578 -> [w606]
              tunnel: [w614] -> w582
              tunnel: w585 -> [w600]
              tunnel: w584 -> [w601]
              frame #0 {
                n260 = Subtract(x=w606, y=w607) -> (x-y=w615:dbl)
                n261 = Add(x=w615, y=1) -> (x+y=w608:dbl)
                n262 = Array Subset(array=w601, index (row)=w607, length (row)=w608) -> (w605:dbl[][])  [unwired: 2 in]
                n263 = Transpose 2D Array(2D array=w605) -> (transposed array=w604:dbl[][])
                n264 = Array Subset(array=w605, index (row)=0, length (row)=w608, index (col)=0, length (col)=w600) -> (w602:dbl[][])
                n265 = Add Array Elements(numeric array=w602) -> (sum=w610:dbl)
                n266 = Divide(x=w610, y=w600) -> (x/y=w609:dbl)
                n267 = for {
                  N: w600 -> [_]
                  tunnel: w604 -> [w626]
                  tunnel: [w620] -> w618 mode=indexing
                  tunnel: w609 -> [w619]
                  i -> [w625]
                  n268 = Array Subset(array=w626, index (row)=w625, length (row)=1) -> (w624:dbl[][])  [unwired: 2 in]
                  n269 = Add Array Elements(numeric array=w624) -> (sum=w622:dbl)
                  n270 = Subtract(x=w622, y=w619) -> (x-y=w621:dbl)
                  n271 = Build Array(w621) -> (w620:dbl[])
                }
                n272 = local read item#15() -> (w603:dbl)
                n273 = Reshape Array(w618, w603, w603) -> (w617:dbl[][])
                "Intensity Graph 6" <- w617
                n274 = call-poly <vilib>:"Array To Matrix.vi"("Real 2D Array"=w617) -> ("Real Matrix"=w613:T1)
                n275 = Transpose 2D Array(2D array=w613) -> (transposed array=w614:T1)
                "px" <- w607
                "px" <- w606
              }
            }
          }
        }
      }
    }
  }
